vi "Repeater.vi"(10 "Finish On":T1, 11 "Node In":refnum<class "bt_Node.lvclass">) -> (3 "Node Out":refnum<class "bt_Node.lvclass">)   [LabVIEW 2021, in "BT.lvlib"]
uses:
  BT.lvlib
  Support/Nodes/abs_Node/bt_Node.lvclass
  Support/Nodes/Decorators/Repeater/Support/Finish On - Type.ctl
  Support/Nodes/Decorators/Repeater/bt_Repeater.lvclass
  C:/Users/Tim/Documents/GitHub/LV_Behaviour_Tree/Source/Support/Nodes/Decorators/abs_Decorator/abs_Decorator.lvclass
  C:/Users/Tim/Documents/GitHub/LV_Behaviour_Tree/Source/Support/Nodes/abs_Node/bt_Node.lvclass
  Support/Nodes/Decorators/Support/Decorator/bt_Decorator.lvclass/bt_Decorator.ctl
  Support/Nodes/Decorators/Repeater/bt_Repeater.lvclass/bt_Repeater.ctl
  Support/Nodes/Decorators/Support/Decorator/Properties/Write Node.vi
  Support/Nodes/Decorators/Repeater/Properties/Write Finish On.vi
  C:/Users/Tim/Documents/GitHub/LV_Behaviour_Tree/Source/Support/Nodes/Decorators/Support/Decorator/bt_Decorator.lvclass
  C:/Users/Tim/Documents/GitHub/LV_Behaviour_Tree/Source/Support/Nodes/Decorators/Repeater/bt_Repeater.lvclass
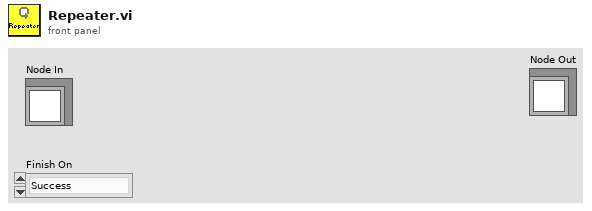
[diagram p1: front panel]
types:
  T1 = typedef "BT.lvlib/bt_Repeater.lvclass/Finish On - Type.ctl" = enum16{"Success", "Failure", "Never"}
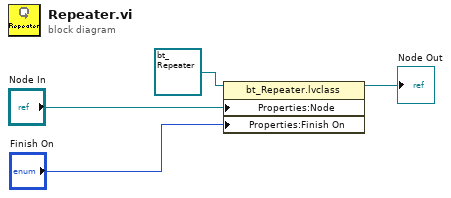
[diagram p0: block diagram]
diagram:
  n1 = property class="bt_Repeater.lvclass"(reference=refnum<class "bt_Repeater.lvclass"> refnum ("BT.lvlib:Repeater.lvclass"), "Properties:Node"="Node In", "Properties:Finish On"="Finish On") -> (reference out=→"Node Out":refnum<class "bt_Repeater.lvclass">)  [unwired: 1 in, 1 out]
